vi "Coord window-Bundle exp params.vi"(11 "Item Names":string[][](array[string])) -> (3 "Item Names + exp params":string[][](array[string]))   [LabVIEW 2013]
uses:
  Global Variables/gl_UI Ctrl Refs.vi
  Globals/Coord window-Globals.vi
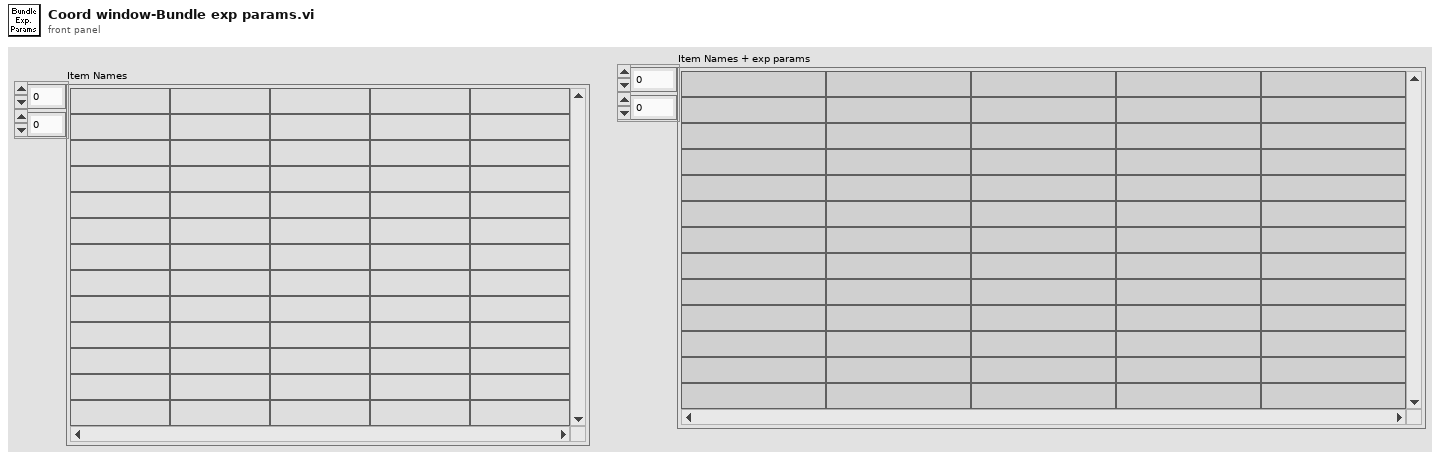
[diagram p1: front panel]
types:
  T1 = typedef "UI ctrl refs cluster.ctl" = cluster{"Top level VI path":path, "Top level VI ref":refnum<vi>, "User menu ref":refnum<k9>, "Sub Panel control":refnum<vi>, "Imaging Param Tab":refnum<vi>, "Occurrence-Start drivers":refnum<k4>, "Occurrence-Speed logging initialised":refnum<k4>, "Occurrence-XYZ stage initialised":refnum<k4>, "Exit button":refnum<vi>, "Status ind":refnum<vi>, "Return to Origin":refnum<vi>, "Speed Logging":refnum<vi>, "Time Lapse":refnum<vi>, "Live Imaging":refnum<vi>, "AOL Z Stack":refnum<vi>, "Motor Z Stack":refnum<vi>, "Funct Acq button":refnum<vi>, "Hard Shutter":refnum<vi>, "Virtual Shutter":refnum<vi>, "Laser Power":refnum<vi>, "AOL Mode":refnum<vi>, "Frame Size":refnum<vi>, "Field of View":refnum<vi>, "Dwell Time":refnum<vi>, "Zoom":refnum<vi>, "AOL Z":refnum<vi>, "Objective":refnum<vi>, "Axis":refnum<vi>, "Paths & Names":refnum<vi>, "Experiment folder path (ind.)":refnum<vi>, "Last State (Ind.)":refnum<vi>, "Laser wavelength ind (nm)":refnum<vi>, "Averages":refnum<vi>, "Angle (degrees)":refnum<vi>, "X centre":refnum<vi>, "Y centre":refnum<vi>, "Plane Mode":refnum<vi>, "# Planes":refnum<vi>, "Z Start":refnum<vi>, "Z Stop":refnum<vi>, "Z Step":refnum<vi>, "PMT 1":refnum<vi>, "PMT 2":refnum<vi>, "Stage XYZ Position":refnum<vi>, "Pockels@Z Start":refnum<vi>, "Pockels@Z Stop":refnum<vi>, "Obtain Z Start":refnum<vi>, "Obtain Z Stop":refnum<vi>, "Live stim.trig.period":refnum<vi>, "Live stim.trig.enable":refnum<vi>, "Funct. Acq. Pockels Modulation":refnum<vi>, "Enable Video Recording":refnum<vi>, "Video Record-Live Imaging":refnum<vi>, "Video Record-Funct acq":refnum<vi>, "AOL Z-stack Chirps Ready (ind)":refnum<vi>, "Center freq ind (nm)":refnum<vi>, "Logging queue (ind)":refnum<vi>, "Back aperture power (ind.)":refnum<vi>, "Power after objective (ind.)":refnum<vi>, "Switch user":refnum<vi>}
  T2 = typedef "Coordinate list window refs.ctl" = cluster{"Window Name (i.e. Key)":string, "menu reference":refnum<k9>, "VI's reference":refnum<vi>, "Pane 1":refnum<vi>, "Pane 2":refnum<vi>, "Coord Listbox":refnum<vi>, "File name":refnum<vi>, "Picture Map":refnum<vi>, "Stage XYZ Position ind.":refnum<vi>}
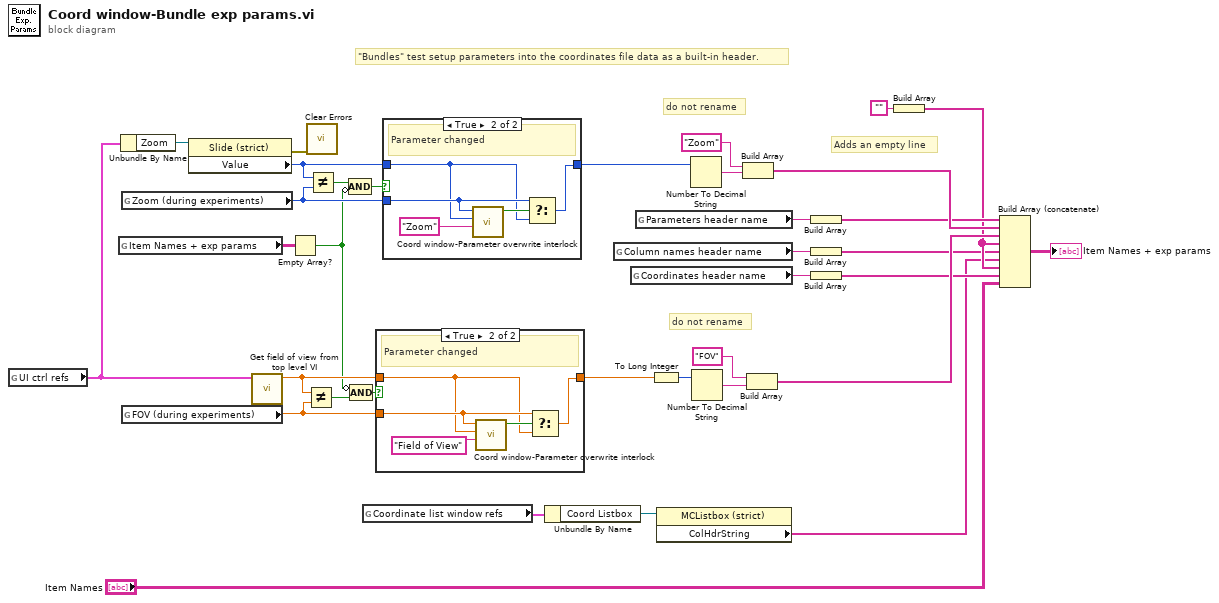
[diagram p0: block diagram]
diagram:
  # "do not rename"
  # "do not rename"
  # "\"Bundles\" test setup parameters into the coordinates file data as a built-in header."
  # "Adds an empty line"
  n1 = global read "gl_UI Ctrl Refs.vi" "UI ctrl refs"() -> (w11:T1)
  n2 = global read "Coord window-Globals.vi" "Item Names + exp params"() -> (w7:string[][])
  n3 = Unbundle By Name(w11) -> ("Zoom"=w35:refnum<vi>)
  n4 = global read "Coord window-Globals.vi" "Zoom (during experiments)"() -> (w20:i8)
  n5 = global read "Coord window-Globals.vi" "FOV (during experiments)"() -> (w15:sgl)
  n6 = property on="Property Node" class="Slide (strict)"(reference=w35) -> (error out=w1:errorcluster, "Value"=w19:i8)  [unwired: 1 in, 1 out]
  n7 = call "Get field of view from top level VI.vi"("UI ctrl refs"=w11) -> ("Field of view (um)"=w16:sgl)  [unwired: 10 in]
  n8 = Empty Array?(array=w7) -> (empty?=w2:bool)
  n9 = Not Equal?(x=w16, y=w15) -> (x != y?=w4:bool)
  n10 = call <vilib>:"Clear Errors.vi"("error in (no error)"=w1) -> ()  [unwired: 6 in, 1 out]
  n11 = Not Equal?(x=w19, y=w20) -> (x != y?=w6:bool)
  n12 = Compound Arithmetic op=AND(w6, invert w2) -> (w5:bool)
  n13 = Compound Arithmetic op=AND(invert w2, w4) -> (w3:bool)
  n14 = global read "Coord window-Globals.vi" "Coordinate list window refs"() -> (w10:T2)
  n15 = case shown="True" w3 {
    tunnel: w15 -> [_ w39]
    tunnel: w16 -> [w36 w37]
    tunnel: [w36 w38] -> w17
    frame False {
      # "No change"
    }
    frame True {
      # "Parameter changed"
      n16 = call "Coord window-Parameter overwrite interlock.vi"("Parameter name"="Field of View", "Parameter's new value"=w37, "Parameter's old value"=w39) -> ("Cancelled"=w41:bool)  [unwired: 8 in]
      n17 = Select(t=w39, s=w41, f=w37) -> (s? t:f=w38:sgl)
    }
  }
  n18 = case shown="True" w5 {
    tunnel: w20 -> [_ w45]
    tunnel: w19 -> [w42 w43]
    tunnel: [w42 w44] -> w18
    frame False {
      # "No change"
    }
    frame True {
      # "Parameter changed"
      n19 = call "Coord window-Parameter overwrite interlock.vi"("Parameter name"="Zoom", "Parameter's new value"=w43, "Parameter's old value"=w45) -> ("Cancelled"=w47:bool)  [unwired: 8 in]
      n20 = Select(t=w45, s=w47, f=w43) -> (s? t:f=w44:i8)
    }
  }
  n21 = Unbundle By Name(w10) -> ("Coord Listbox"=w9:refnum<vi>)
  n22 = global read "Coord window-Globals.vi" "Column names header name"() -> (w13:string)
  n23 = global read "Coord window-Globals.vi" "Coordinates header name"() -> (w22:string)
  n24 = global read "Coord window-Globals.vi" "Parameters header name"() -> (w21:string)
  n25 = To Long Integer(number=w17) -> (32bit integer=w34:i32)
  n26 = property on="Property Node" class="MCListbox (strict)"(reference=w9) -> ("ColHdrString"=w8:string[])  [unwired: 1 in, 2 out]
  n27 = Number To Decimal String(number=w18) -> (decimal integer string=w32:string)  [unwired: 1 in]
  n28 = Number To Decimal String(number=w34) -> (decimal integer string=w29:string)  [unwired: 1 in]
  n29 = Build Array("Zoom", w32) -> (w31:string[])
  n30 = Build Array("FOV", w29) -> (w28:string[])
  n31 = Build Array(w21) -> (w26:string[])
  n32 = Build Array(w13) -> (w12:string[])
  n33 = Build Array(w22) -> (w25:string[])
  n34 = Build Array("") -> (w14:string[])
  n35 = Build Array (concatenate)(w26, w31, w28, w14, w12, w8, w14, w25, "Item Names") -> (→"Item Names + exp params":string[][])
